vi "CRYMake Generator Index.vi"() -> (3 "Gen_Index":i32)   [LabVIEW 2013]
uses:
  CRYMisc vis settings global.vi
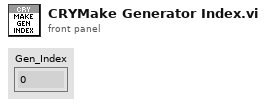
[diagram p1: front panel]
types:
  T1 = cluster{"Gen Idx":i32, "Chn Idx":i32, "Data":sgl[]}[]
  T2 = cluster{"Gen Idx":i32, "Chn Idx":i32, "Data":i32[]}
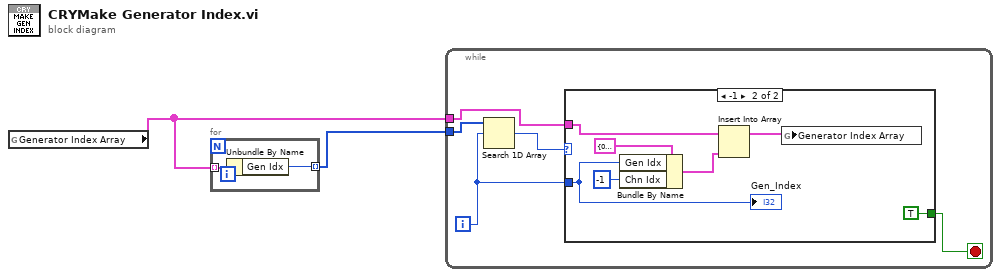
[diagram p0: block diagram]
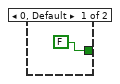
[diagram p2: hidden frame]
diagram:
  n1 = global read "CRYMisc vis settings global.vi" "Generator Index Array"() -> (w2:T1)
  n2 = for {
    tunnel: w2 -> [w4] mode=indexing
    tunnel: [w3] -> w1 mode=indexing
    n3 = Unbundle By Name(w4) -> ("Gen Idx"=w3:i32)
  }
  n4 = while {
    tunnel: w2 -> [w5]
    tunnel: w1 -> [w6]
    i -> [w8]
    stop <- w7 stop-if-true
    n5 = Search 1D Array(1D array=w6, element=w8) -> (index of element=w9:i32)  [unwired: 1 in]
    n6 = case shown="-1" w9 {
      tunnel: [FALSE TRUE] -> w7
      tunnel: w5 -> [_ w16]
      tunnel: w8 -> [_ w14]
      frame 0, Default {
      }
      frame -1 {
        n7 = Bundle By Name(cluster=T2 {"Gen Idx"=0, "Chn Idx"=0, "Data"=[]} ("Cluster"), "Gen Idx"=w14, "Chn Idx"=-1) -> (w12:T2)
        n8 = Insert Into Array(array=w16, new element=w12) -> (w15:T1)  [unwired: 1 in]
        n9 = global write "CRYMisc vis settings global.vi" "Generator Index Array"(w15) -> ()
        "Gen_Index" <- w14
      }
    }
  }
